vi "Test Audio Streamer.vi"() -> ()   [LabVIEW 2020]
uses:
  Typedefs/AudioStreamer.Config Return Data.ctl
  Typedefs/AudioStreamer.Globals.vi
  <vilib>/Analysis/NI_AALBase.lvlib
panel:
  out "config":T1
  in  "OK Button":bool
  out "trig":bool
  out "streamer is open":bool
  out "Error message":string
  out "Status":string
  in  "Stop":bool
  in  "Start":bool
  in  "Trigger":bool
  out "Waveform Graph":dbl[][](graph)
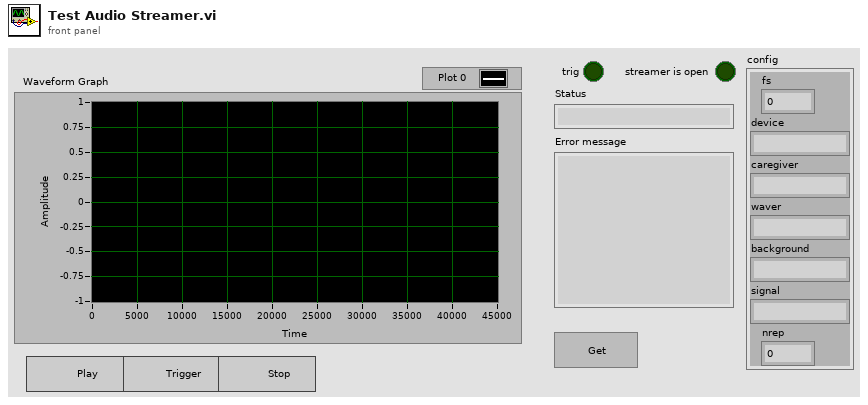
[diagram p1: front panel]
types:
  T1 = typedef "AudioStreamer.Config Return Data.ctl" = cluster{"fs":dbl, "device":string, "caregiver":string, "waver":string, "background":string, "signal":string, "nrep":i32}
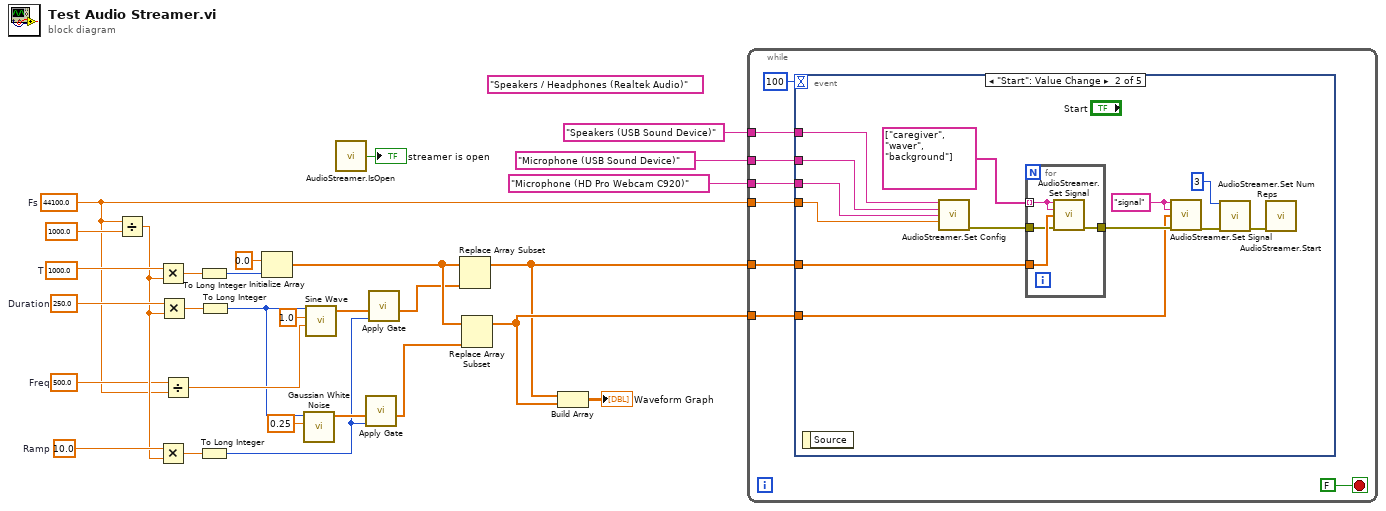
[diagram p0: block diagram]
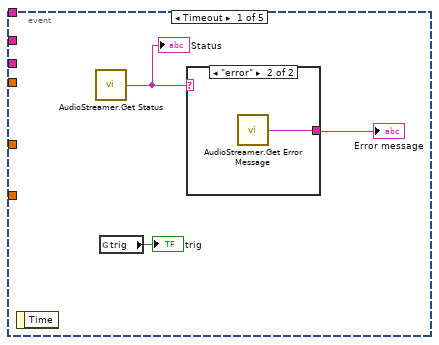
[diagram p2: hidden frame]
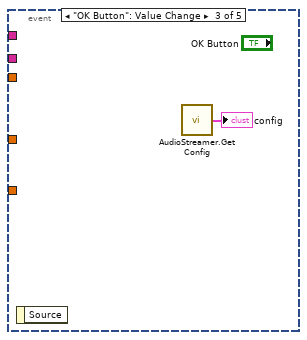
[diagram p4: hidden frame]
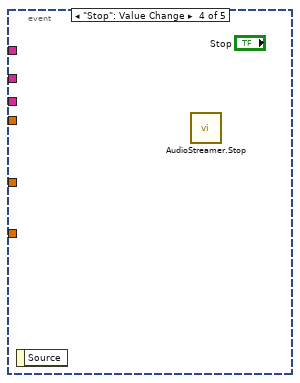
[diagram p5: hidden frame]
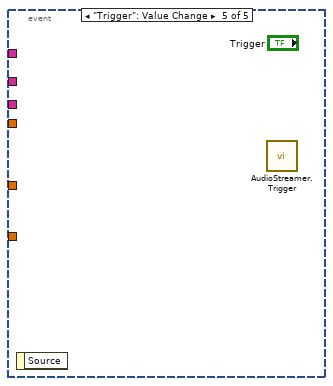
[diagram p6: hidden frame]
diagram:
  (unwired) "Speakers / Headphones (Realtek Audio)"
  w18 = 500.0  # Freq
  w23 = 10.0  # Ramp
  w25 = 250.0  # Duration
  w28 = 1000.0  # T
  w9 = 44100.0  # Fs
  n1 = Divide(x=w9, y=1000.0) -> (x/y=w22:dbl)
  n2 = Multiply(x=w28, y=w22) -> (x*y=w27:dbl)
  n3 = Multiply(x=w23, y=w22) -> (x*y=w24:dbl)
  n4 = Multiply(x=w25, y=w22) -> (x*y=w26:dbl)
  n5 = Divide(x=w18, y=w9) -> (x/y=w17:dbl)
  n6 = To Long Integer(number=w27) -> (32bit integer=w21:i32)
  n7 = To Long Integer(number=w24) -> (32bit integer=w12:i32)
  n8 = To Long Integer(number=w26) -> (32bit integer=w16:i32)
  n9 = Initialize Array(0.0 ("element"), w21) -> (w15:dbl[])
  n10 = call <vilib>:"Gaussian White Noise.vi"("standard deviation"=0.25, "samples"=w16) -> ("Gaussian noise pattern"=w13:dbl[])  [unwired: 8 in, 1 out]
  n11 = call <vilib>:"Sine Wave.vi"("samples"=w16, "amplitude"=1.0, "frequency"=w17) -> ("sine wave"=w14:dbl[])  [unwired: 2 in, 2 out]
  n12 = call "AudioStreamer.IsOpen.vi"() -> ("success"=→"streamer is open":bool)  [unwired: 1 in]
  n13 = call "Apply Gate.vi"("nramp"=w12, "Waveform in"=w13) -> ("Gated waveform"=w6:dbl[])  [unwired: 9 in]
  n14 = call "Apply Gate.vi"("nramp"=w12, "Waveform in"=w14) -> ("Gated waveform"=w7:dbl[])  [unwired: 9 in]
  n15 = Replace Array Subset(array=w15, new element=w7) -> (w8:dbl[])  [unwired: 1 in]
  n16 = Replace Array Subset(array=w15, new element=w6) -> (w10:dbl[])  [unwired: 1 in]
  n17 = Build Array(w8, w10) -> (→"Waveform Graph":dbl[][])
  n18 = while {
    tunnel: w8 -> [w36]
    tunnel: w10 -> [w35]
    tunnel: w9 -> [w33]
    tunnel: "Speakers (USB Sound Device)" -> [w32]
    tunnel: "Microphone (USB Sound Device)" -> [w31]
    tunnel: "Microphone (HD Pro Webcam C920)" -> [w30]
    stop <- FALSE stop-if-true
    n19 = event shown="[1] \"Start\": Value Change" {
      selector: _ -> [_ _ _ _ _]
      dyn-events: _ -> [_ _ _ _ _]
      timeout: 100 -> [_ _ _ _ _]
      tunnel: w36 -> [_ w53 _ _ _]
      tunnel: w35 -> [_ w50 _ _ _]
      tunnel: w33 -> [_ w44 _ _ _]
      tunnel: w32 -> [_ w46 _ _ _]
      tunnel: w31 -> [_ w45 _ _ _]
      tunnel: w30 -> [_ w43 _ _ _]
      event Timeout {
        n20 = event-data() -> ()  [unwired: 1 in, 1 out]
        n21 = call "AudioStreamer.Get Status.vi"() -> ("status"=w40:string)  [unwired: 1 in]
        "Status" <- w40
        n22 = global read "AudioStreamer.Globals.vi" "trig"() -> (→"trig":bool)
        n23 = case shown="\"error\"" w40 {
          tunnel: [_ w41] -> w39
          frame "", Default {
          }
          frame "error" {
            n24 = call "AudioStreamer.Get Error Message.vi"() -> ("message"=w41:string)  [unwired: 1 in]
          }
        }
        "Error message" <- w39
      }
      event "Start": Value Change {
        w42 = "signal" ("destination")
        n25 = event-data() -> ()  [unwired: 1 in, 1 out]
        n26 = call "AudioStreamer.Set Config.vi"("output"=w46, "mic"=w45, "waverMic"=w43, "Fs (Hz)"=w44) -> ("error out"=w52:errorcluster)  [unwired: 11 in]
        n27 = for {
          tunnel: string[] ["caregiver", "waver", "background"] -> [w55] mode=indexing
          tunnel: w53 -> [w58]
          tunnel: w52 -> [w57]
          tunnel: [w56] -> w51
          n28 = call "AudioStreamer.Set Signal.vi"("destination"=w55, "name"=w55, "data"=w58, "error in (no error)"=w57) -> ("error out"=w56:errorcluster)  [unwired: 11 in]
        }
        n29 = call "AudioStreamer.Set Signal.vi"("destination"=w42, "name"=w42, "data"=w50, "error in (no error)"=w51) -> ("error out"=w49:errorcluster)  [unwired: 11 in]
        n30 = call "AudioStreamer.Set Num Reps.vi"("nreps"=3, "error in (no error)"=w49) -> ("error out"=w48:errorcluster)  [unwired: 13 in]
        n31 = call "AudioStreamer.Start.vi"("error in (no error)"=w48) -> ()  [unwired: 14 in, 1 out]
      }
      event "OK Button": Value Change {
        n32 = event-data() -> ()  [unwired: 1 in, 1 out]
        n33 = call "AudioStreamer.Get Config.vi"() -> ("config"=→"config":T1)  [unwired: 1 in]
      }
      event "Stop": Value Change {
        n34 = event-data() -> ()  [unwired: 1 in, 1 out]
        n35 = call "AudioStreamer.Stop.vi"() -> ()  [unwired: 15 in, 1 out]
      }
      event "Trigger": Value Change {
        n36 = event-data() -> ()  [unwired: 1 in, 1 out]
        n37 = call "AudioStreamer.Trigger.vi"() -> ()  [unwired: 15 in, 1 out]
      }
    }
  }
